vi "FGV_HovaCAL_Interface_ControlReferenzen.vi"(6 "Aktion":enum16{"lesen", "schreiben"}(ring), 7 "MFC fix Cluster":T2, 8 "Fehler (Eingang, kein Fehler)":errorcluster, 9 "System Cluster":T5, 10 "Set Cluster":T4, 11 "Get Cluster":T1) -> (0 "Fehler (Ausgang)":errorcluster, 1 "System Cluster out":T5, 2 "Set Cluster out":T3, 3 "Get Cluster out":T1, 5 "MFC fix Cluster out":T2)   [LabVIEW 2020, in "Linearisierung v2.lvlib" / "Gasteiler.lvlib" / "HovaCAL_Interface.lvlib" / "Kommunikation.lvlib"]
uses:
  Kommunikation.lvlib
  Controls/MFC Einstellungen.ctl
  Controls/Controls.lvlib
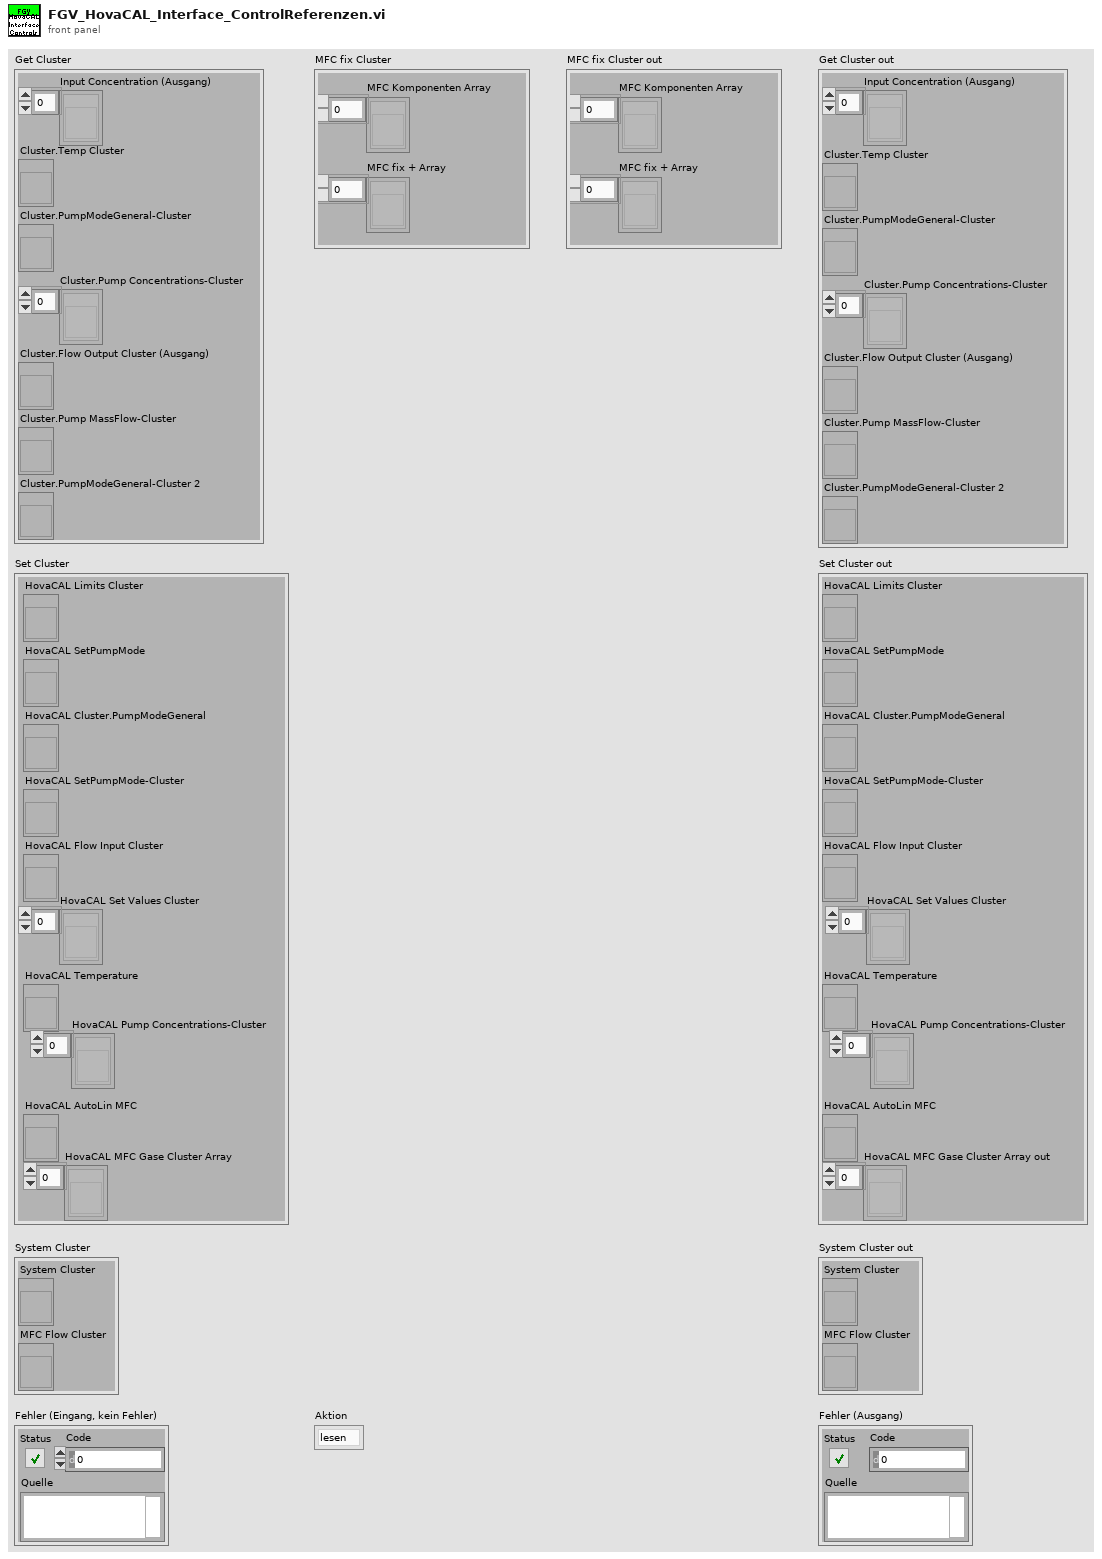
[diagram p1: front panel]
types:
  T1 = cluster{"Input Concentration (Ausgang)":refnum<vi>[], "Cluster.Temp Cluster":refnum<vi>, "Cluster.PumpModeGeneral-Cluster":refnum<vi>, "Cluster.Pump Concentrations-Cluster":refnum<vi>[], "Cluster.Flow Output Cluster (Ausgang)":refnum<vi>, "Cluster.Pump MassFlow-Cluster":refnum<vi>, "Cluster.PumpModeGeneral-Cluster 2":refnum<vi>}
  T2 = cluster{"MFC Komponenten Array":refnum<vi>[], "MFC fix + Array":refnum<vi>[]}
  T3 = cluster{"HovaCAL Limits Cluster":refnum<vi>, "HovaCAL SetPumpMode":refnum<vi>, "HovaCAL Cluster.PumpModeGeneral":refnum<vi>, "HovaCAL SetPumpMode-Cluster":refnum<vi>, "HovaCAL Flow Input Cluster":refnum<vi>, "HovaCAL Set Values Cluster":refnum<vi>[], "HovaCAL Temperature":refnum<vi>, "HovaCAL Pump Concentrations-Cluster":refnum<vi>[], "HovaCAL AutoLin MFC":refnum<vi>, "HovaCAL MFC Gase Cluster Array out":refnum<vi>[]}
  T4 = cluster{"HovaCAL Limits Cluster":refnum<vi>, "HovaCAL SetPumpMode":refnum<vi>, "HovaCAL Cluster.PumpModeGeneral":refnum<vi>, "HovaCAL SetPumpMode-Cluster":refnum<vi>, "HovaCAL Flow Input Cluster":refnum<vi>, "HovaCAL Set Values Cluster":refnum<vi>[], "HovaCAL Temperature":refnum<vi>, "HovaCAL Pump Concentrations-Cluster":refnum<vi>[], "HovaCAL AutoLin MFC":refnum<vi>, "HovaCAL MFC Gase Cluster Array":refnum<vi>[]}
  T5 = cluster{"System Cluster":refnum<vi>, "MFC Flow Cluster":refnum<vi>}
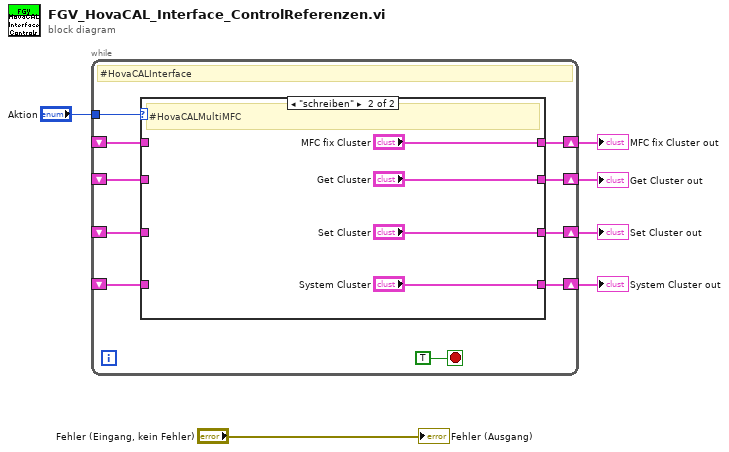
[diagram p0: block diagram]
diagram:
  n1 = while {
    tunnel: "Aktion" -> [w15]
    shift-right: [w14] -> w1
    shift-left: _ -> [w12]
    shift-right: [w13] -> w5
    shift-left: _ -> [w11]
    shift-right: [w10] -> w4
    shift-left: _ -> [w9]
    shift-right: [w8] -> w2
    shift-left: _ -> [w7]
    stop <- TRUE stop-if-true
    # "#HovaCALInterface"
    n2 = case shown="\"schreiben\"" w15 {
      tunnel: [w20 "Get Cluster"] -> w14
      tunnel: [w19 "Set Cluster"] -> w13
      tunnel: w12 -> [w20 _]
      tunnel: w11 -> [w19 _]
      tunnel: [w18 "System Cluster"] -> w10
      tunnel: w9 -> [w18 _]
      tunnel: [w17 "MFC fix Cluster"] -> w8
      tunnel: w7 -> [w17 _]
      frame "lesen", Default {
        # "#HovaCALMultiMFC"
      }
      frame "schreiben" {
        # "#HovaCALMultiMFC"
      }
    }
  }
  "System Cluster out" <- w4
  "Set Cluster out" <- w5
  "MFC fix Cluster out" <- w2
  "Get Cluster out" <- w1
  "Fehler (Ausgang)" <- "Fehler (Eingang, kein Fehler)"
